vi "Get Field Path.vi"() -> (3 "appended path":path)   [LabVIEW 2015]
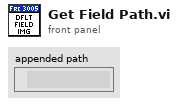
[diagram p1: front panel]
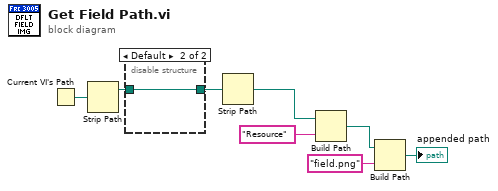
[diagram p0: block diagram]
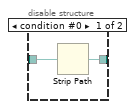
[diagram p2: hidden frame]
diagram:
  n1 = Current VI's Path() -> (path=w4:path)
  n2 = Strip Path(path=w4) -> (stripped path=w3:path)  [unwired: 1 out]
  n3 = disable-structure shown="Default" {
    disable-tunnel: w3 -> [w10 w11]
    disable-tunnel: [w9 w11] -> w1
    frame condition #0 {
      n4 = Strip Path(path=w10) -> (stripped path=w9:path)  [unwired: 1 out]
    }
    frame condition #1 (active) {
    }
  }
  n5 = Strip Path(path=w1) -> (stripped path=w2:path)  [unwired: 1 out]
  n6 = Build Path(base path=w2, name or relative path="Resource") -> (appended path=w7:path)
  n7 = Build Path(base path=w7, name or relative path="field.png") -> (appended path=→"appended path":path)
